vi "Get Package Names and Versions.vi"(11 "NIPKG Result":string) -> (3 "Packages":string[][](table))   [LabVIEW 2014, in "NIPM_API.lvlib"]
doc: "Parses the NIPGK command's response to get the list of Package Names and Versions\n\nINPUT(s)\n<B>NIPKG Result</B>: This is the string output from a NIPKG command that contains pacakges names, version, and single line description.\n\nOUTPUT(s)\n<B>Packages</B>: List of package names and their version as a 2D string array"
uses:
  NIPM_API.lvlib
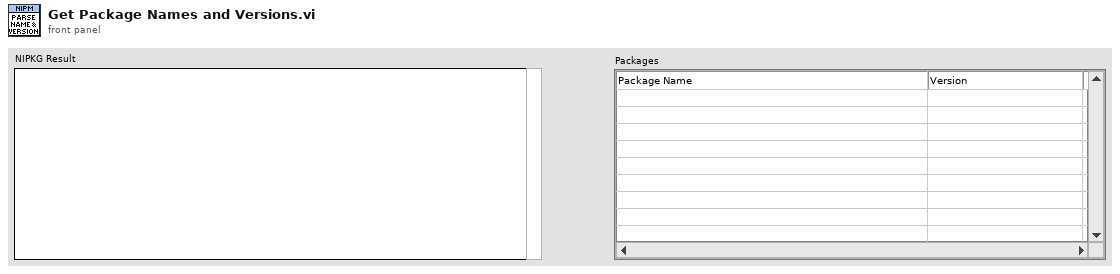
[diagram p1: front panel]
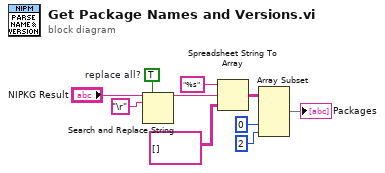
[diagram p0: block diagram]
diagram:
  w6 = TRUE  # replace all?
  n1 = Search and Replace String(replace all?=w6, input string="NIPKG Result", search string="\r") -> (result string=w8:string)  [unwired: 5 in, 3 out]
  n2 = Spreadsheet String To Array(format string="%s", spreadsheet string=w8, array type (2D Dbl)=string[][] []) -> (array=w5:string[][])  [unwired: 1 in]
  n3 = Array Subset(array=w5, index (col)=0 ("disabled index (col)"), length (col)=2 ("length")) -> (→"Packages":string[][])  [unwired: 2 in]
